vi "FFT_based_prediction_Computationtime_v2.vi"() -> ()   [LabVIEW 2020]
uses:
  <vilib>/Utility/file.llb/Read Delimited Spreadsheet (DBL).vi
panel:
  out "x-y":u32
  out "Frequency Interval: delta(f) 3":dbl
  out "xf (frequency) 3":dbl[](array[numeric])
  out "size(s) 3":i32
  out "df (Hz) 3":dbl
  out "Time vs Acceleration ( Input learning length) 2":cluster{dbl[], dbl[]}[](graph)
  out "array w/ subset deleted 3":dbl[][](array[numeric])
  out "time 3":dbl[](array[numeric])
  out "Acceleration 3":dbl[](array[numeric])
  out "Time vs Acceleration graph(whole data)  2":cluster{"all rows":dbl[], "all rows":dbl[]}(graph)
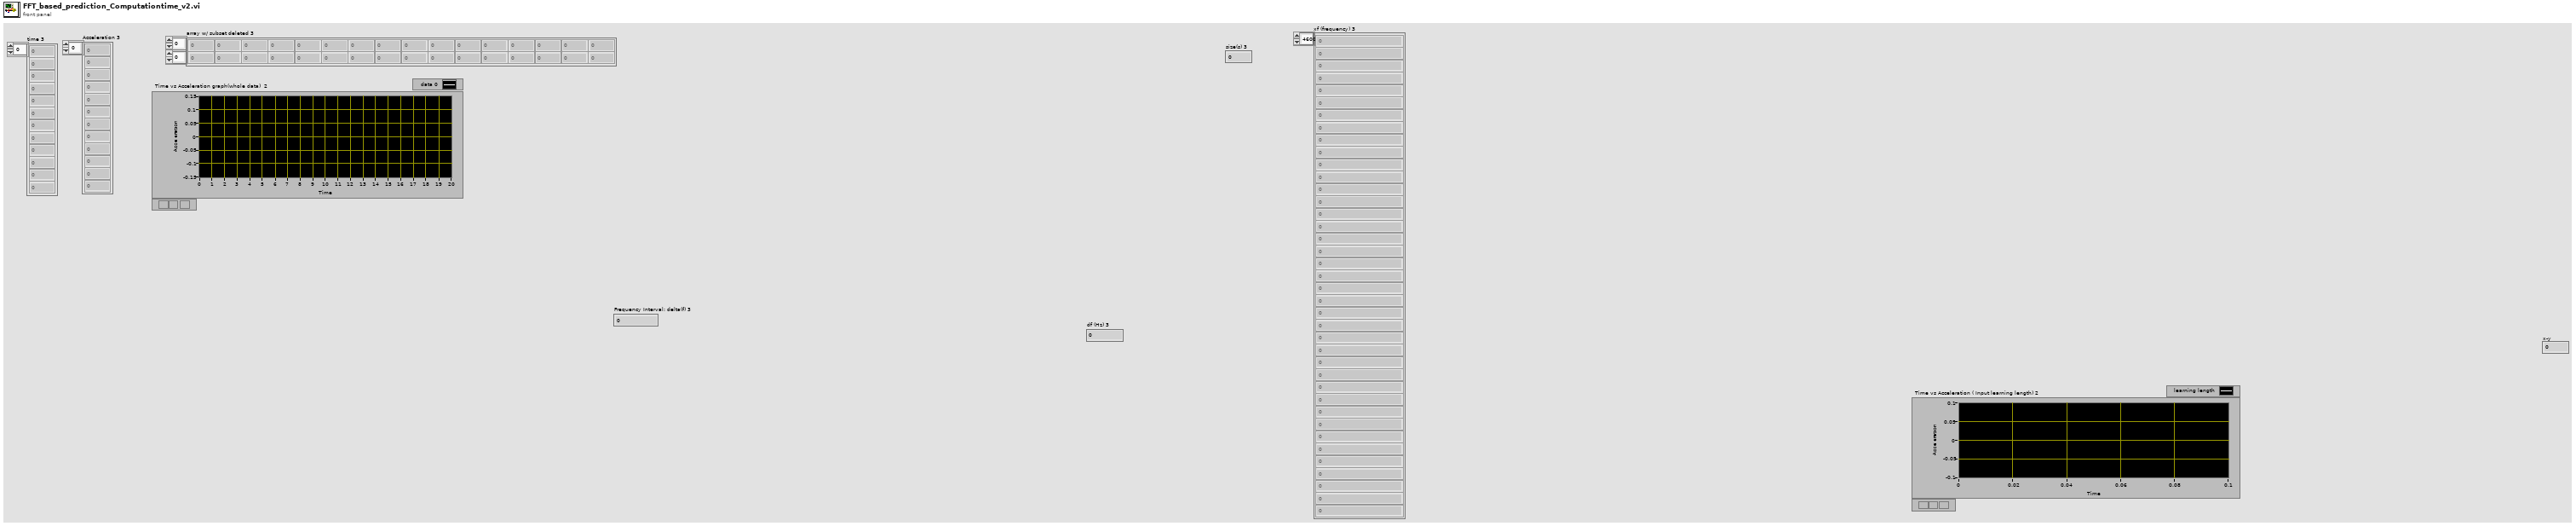
[diagram p1: front panel]
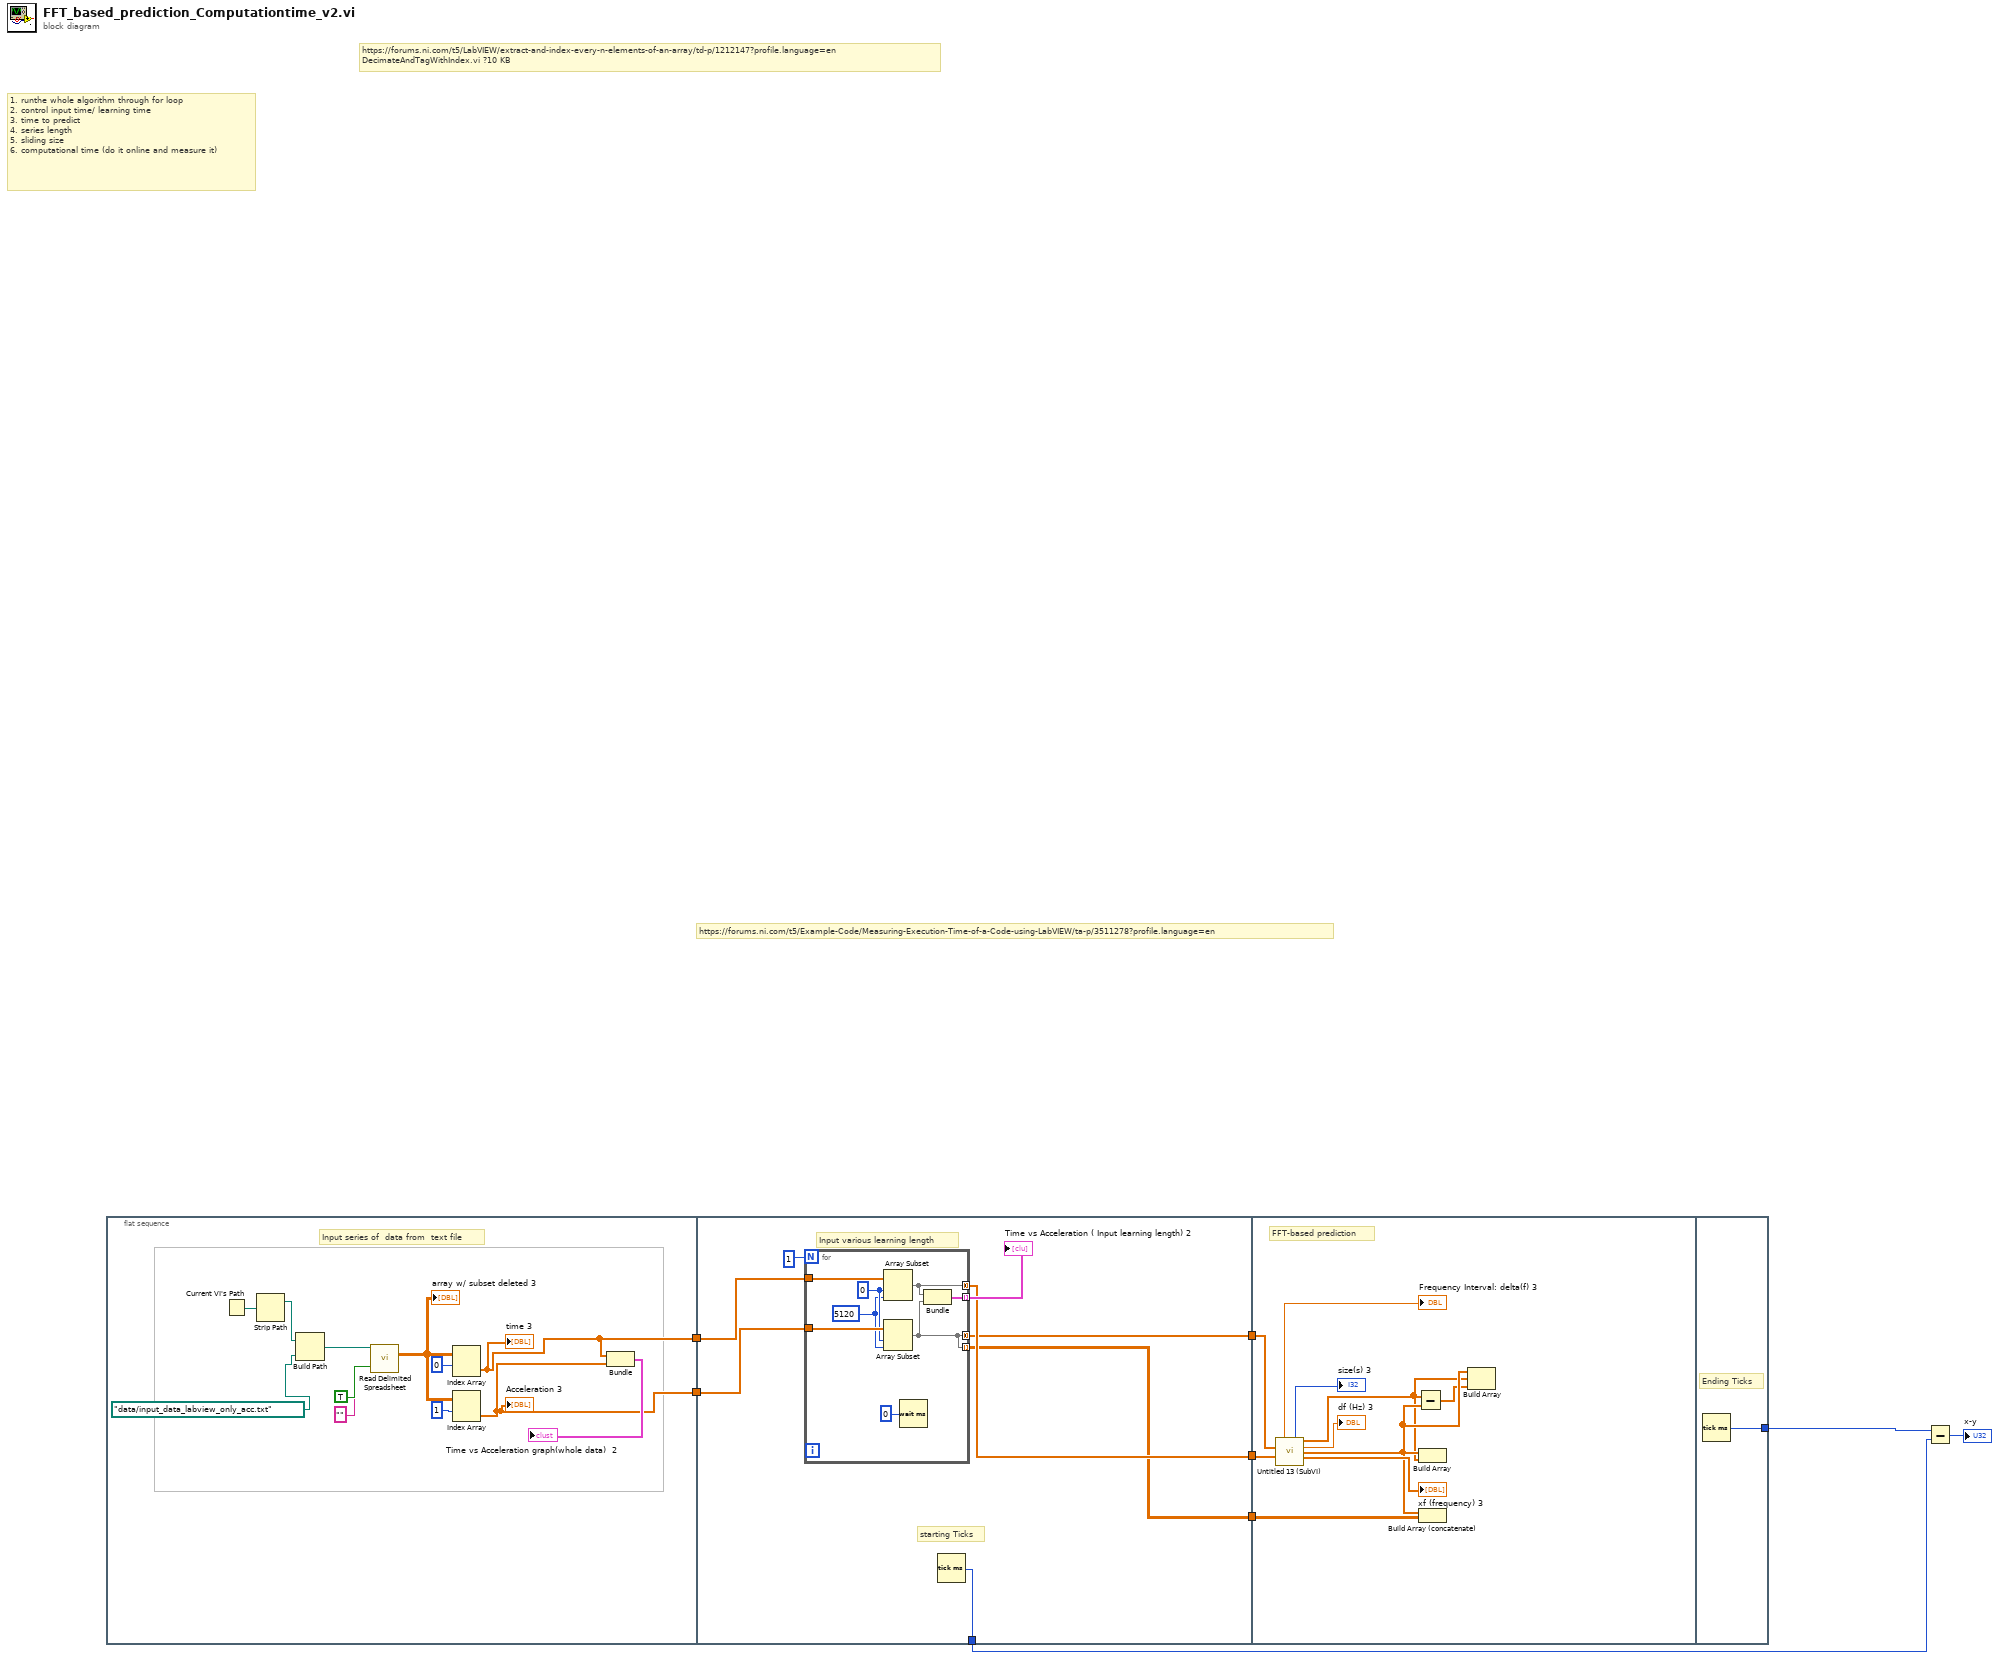
[diagram p0: block diagram]
diagram:
  # "https://forums.ni.com/t5/Example-Code/Measuring-Execution-Time-of-a-Code-using-LabVIEW/ta-p/3511278?profile.language=en"
  # "1. runthe whole algorithm through for loop \n2. control input time/ learning time\n3. time to predict\n4. series length\n5. sliding size\n6. computational time (do it online and measure it)"
  # "https://forums.ni.com/t5/LabVIEW/extract-and-index-every-n-elements-of-an-array/td-p/1212147?profile.language=en\nDecimateAndTagWithIndex.vi ?10 KB"
  n1 = flat-sequence {
    tunnel: [w11] -> w8
    tunnel: [w10] -> w7
    tunnel: w8 -> [w27]
    tunnel: w7 -> [w26]
    tunnel: [w24] -> w6
    tunnel: [w23] -> w5
    tunnel: [w22] -> w4
    tunnel: [w21] -> w1
    tunnel: w6 -> [w39]
    tunnel: w5 -> [w38]
    tunnel: w4 -> [w37]
    tunnel: [w47] -> w3
    frame #0 {
      # "Input series of  data from  text file"
      n2 = Current VI's Path() -> (path=w18:path)
      n3 = Strip Path(path=w18) -> (stripped path=w19:path)  [unwired: 1 out]
      n4 = Build Path(base path=w19, name or relative path=path "data/input_data_labview_only_acc.txt") -> (appended path=w20:path)
      n5 = call-poly <vilib>:"Read Delimited Spreadsheet.vi"("file path (dialog if empty)"=w20, "transpose? (F)"=TRUE, "delimiter (\\t)"="" ("delimiter (\\t)")) -> ("all rows"=w17:dbl[][])  [unwired: 7 in, 5 out]
      "array w/ subset deleted 3" <- w17
      n6 = Index Array(array=w17, index (row)=0) -> (element=w11:dbl[])  [unwired: 1 in]
      "time 3" <- w11
      n7 = Index Array(array=w17, index (row)=1) -> (element=w10:dbl[])  [unwired: 1 in]
      "Acceleration 3" <- w10
      n8 = Bundle("all rows"=w11, "all rows"=w10) -> (→"Time vs Acceleration graph(whole data)  2":cluster{"all rows":dbl[], "all rows":dbl[]})  [unwired: 1 in]
    }
    frame #1 {
      # "starting Ticks"
      # "Input various learning length"
      n9 = for {
        N: 1 -> [_]
        tunnel: w27 -> [w36]
        tunnel: [w33] -> w24 mode=concatenating
        tunnel: w26 -> [w35]
        tunnel: [w31] -> w23 mode=concatenating
        tunnel: [w32] -> w25 mode=indexing
        tunnel: [w31] -> w22 mode=indexing
        w34 = 0
        w30 = 5120 ("length")
        n10 = Array Subset(array=w36, index=w34, length=w30) -> (w33:dbl[])
        n11 = Array Subset(array=w35, index=w34, length=w30) -> (w31:dbl[])
        n12 = Wait (ms)(milliseconds to wait=u32 0) -> ()  [unwired: 1 out]
        n13 = Bundle(w33, w31) -> (w32:cluster{dbl[], dbl[]})  [unwired: 1 in]
      }
      "Time vs Acceleration ( Input learning length) 2" <- w25
      n14 = Tick Count (ms)() -> (millisecond timer value=w21:u32)
    }
    frame #2 {
      # "FFT-based prediction"
      n15 = call "Untitled 13 (SubVI).vi"("time"=w39, "acceleration"=w38) -> ("Frequency Interval: delta(f)"=→"Frequency Interval: delta(f) 3":dbl, "size(s)"=→"size(s) 3":i32, "all rows"=w41:dbl[], "df (Hz)"=→"df (Hz) 3":dbl, "Array"=w42:dbl[], "xf (frequency)"=→"xf (frequency) 3":dbl[])  [unwired: 6 in, 2 out]
      n16 = Subtract(x=w41, y=w42) -> (x-y=w40:dbl[])
      n17 = Build Array(w42, w41) -> ()  [unwired: 1 out]
      n18 = Build Array (concatenate)(w42, w37) -> ()  [unwired: 1 out]
      n19 = Build Array(w42, w41, w40) -> ()  [unwired: 1 out]
    }
    frame #3 {
      # "Ending Ticks"
      n20 = Tick Count (ms)() -> (millisecond timer value=w47:u32)
    }
  }
  n21 = Subtract(x=w3, y=w1) -> (x-y=→"x-y":u32)
